vi "send_angles.vi"(7 "url":string, 8 "error in (no error)":errorcluster, 10 "angles and speed":T2={"degrees"=[0.0, 0.0, 0.0, 0.0, 0.0, 0.0], "speed"=30}, 11 "client handle":T1) -> (0 "error out":errorcluster, 3 "client handle out":T1)   [LabVIEW 2022 SP3]
uses:
  angle_speed_def.ctl
  <vilib>/httpClient/PUTBuffer.vi
  <vilib>/httpClient/LabVIEWHTTPClient.lvlib
  <vilib>/httpClient/ClientHandle.ctl
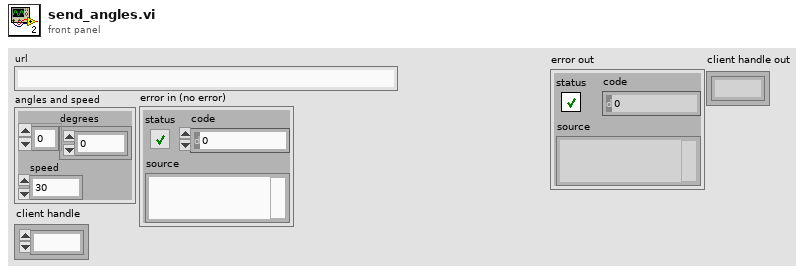
[diagram p1: front panel]
types:
  T1 = typedef "LabVIEWHTTPClient.lvlib/ClientHandle.ctl" = refnum<k1>
  T2 = typedef "angle_speed_def.ctl" = cluster{"degrees":dbl[], "speed":i32}
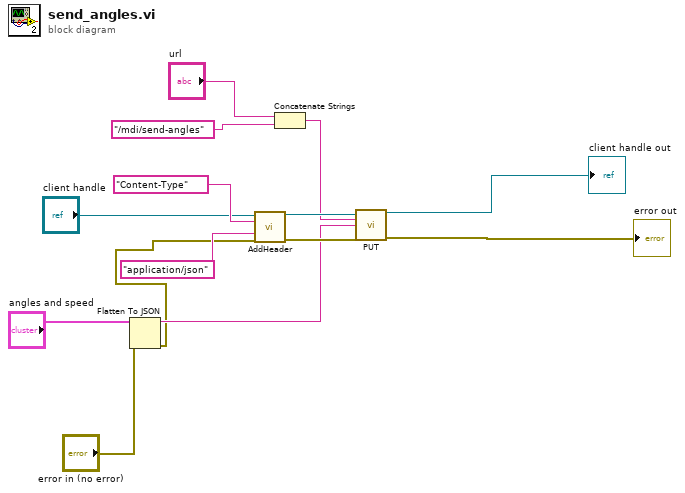
[diagram p0: block diagram]
diagram:
  n1 = Flatten To JSON(anything="angles and speed", error in (no error)="error in (no error)") -> (JSON string=w8:string, 11:w2:errorcluster)  [unwired: 1 in]
  n2 = call <vilib>:"AddHeader.vi"("client handle"="client handle", "header"="Content-Type", "value"="application/json", "error in (no error)"=w2) -> ("client handle out"=w12:T1, "error out"=w13:errorcluster)  [unwired: 10 in]
  n3 = Concatenate Strings("url", "/mdi/send-angles" ("string")) -> (w5:string)
  n4 = call-poly <vilib>:"PUT.vi"("client handle"=w12, "url"=w5, "buffer"=w8, "error in (no error)"=w13) -> ("client handle out"=→"client handle out":T1, "error out"=→"error out":errorcluster)  [unwired: 8 in, 2 out]
